vi "Sequence.FormatConditions.vi"(4 "Aliases.All":T3[](array[typedef]), 6 "Aliases Array":string[](array[string]), 8 "error in (no error)":errorcluster, 10 "Conditions":string[](array[string]), 11 "variant in":variant) -> (0 "error out":errorcluster, 1 "Warning":string, 2 "Condition":T1={"First Opreation"=enum."||", "Expression"=""}, 3 "variant out":variant)   [LabVIEW 2015, in "Simple Sequence Tools - Editor.lvlib"]
uses:
  Simple Sequence Tools - Editor.lvlib
  Shared/Types/Channel.Properties.ctl
  Types/Compiled.StepCondition.ctl
  Types/Conditions.OperationTypes.ctl
  NationalInstruments.VeriStand.RealTimeSequenceDefinitionApiUtilities
  Shared/Simple Sequence Tools - Shared.lvlib
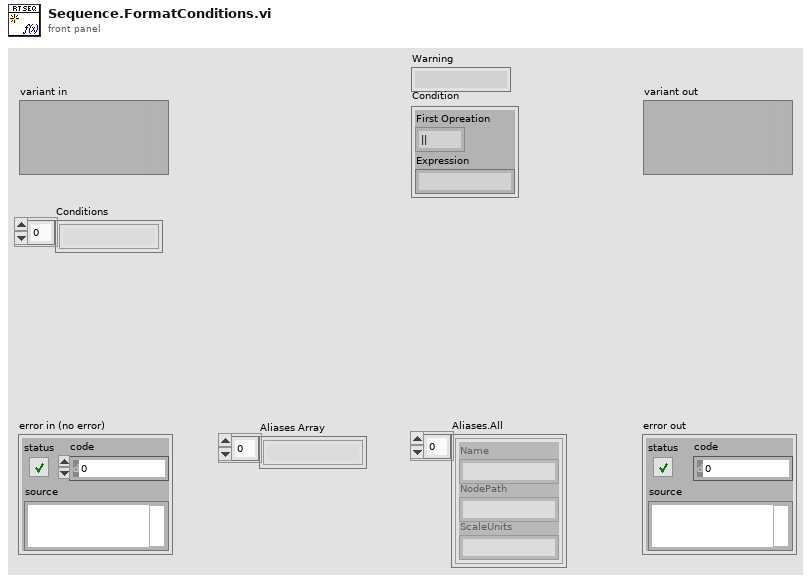
[diagram p1: front panel]
types:
  T1 = typedef "Simple Sequence Tools - Editor.lvlib/Compiled.StepCondition.ctl" = cluster{"First Opreation":T2, "Expression":string}
  T2 = typedef "Simple Sequence Tools - Editor.lvlib/Conditions.OperationTypes.ctl" = enum8{"None", "&&", "||"}
  T3 = typedef "Simple Sequence Tools - Shared.lvlib/Channel.Properties.ctl" = cluster{"Name":string, "NodePath":string, "ScaleUnits":string}
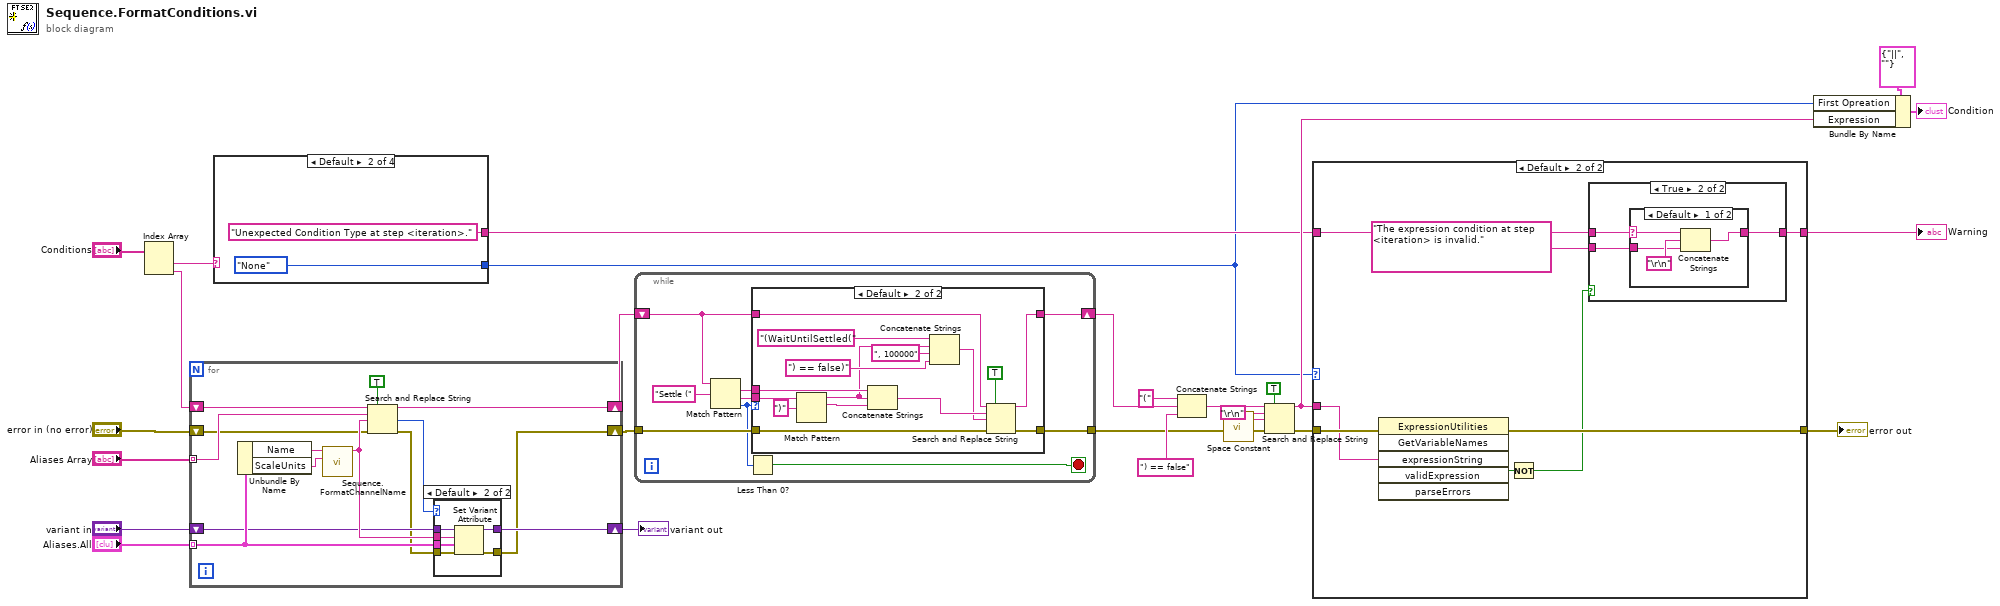
[diagram p0: block diagram]
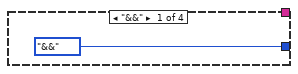
[diagram p7: hidden frame]
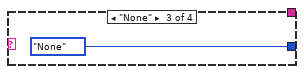
[diagram p8: hidden frame]
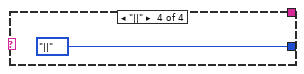
[diagram p9: hidden frame]
diagram:
  n1 = Index Array(array="Conditions") -> (element #1=w15:string, element #2=w14:string)  [unwired: 2 in]
  n2 = for {
    tunnel: "Aliases Array" -> [w40] mode=indexing
    tunnel: "Aliases.All" -> [w34] mode=indexing
    shift-right: [w27] -> w3
    shift-left: "error in (no error)" -> [w31]
    shift-right: [w35] -> w4
    shift-left: w14 -> [w39]
    shift-right: [w32] -> w26
    shift-left: "variant in" -> [w29]
    n3 = Unbundle By Name(w34) -> ("Name"=w37:string, "ScaleUnits"=w38:string)
    n4 = call "Sequence.FormatChannelName.vi"("ScaleUnits"=w38, "Name"=w37) -> ("ChannelName"=w33:string)  [unwired: 9 in]
    n5 = Search and Replace String(replace all?=TRUE ("replace all? (F)"), input string=w39, search string=w40, replace string=w33, error in=w31) -> (result string=w35:string, number of replacements=w30:i32, error out=w28:errorcluster)  [unwired: 3 in, 1 out]
    n6 = case shown="Default" w30 {
      tunnel: w34 -> [_ w48]
      tunnel: w33 -> [_ w47]
      tunnel: [w42 w46] -> w32
      tunnel: w29 -> [w42 w45]
      tunnel: w28 -> [w41 w44]
      tunnel: [w41 w43] -> w27
      frame -1, 0 {
      }
      frame Default {
        n7 = Set Variant Attribute(Variant=w45, name=w47, value=w48, error in=w44) -> (Variant out=w46:variant, error out=w43:errorcluster)  [unwired: 1 out]
      }
    }
  }
  "variant out" <- w26
  n8 = case shown="Default" w15 {
    tunnel: [Conditions.OperationTypes."&&" Conditions.OperationTypes."None" Conditions.OperationTypes."None" Conditions.OperationTypes."||"] -> w6
    tunnel: [_ "Unexpected Condition Type at step <iteration>." _ _] -> w8
    frame "&&" {
    }
    frame Default {
    }
    frame "None" {
    }
    frame "||" {
    }
  }
  n9 = while {
    shift-right: [w58] -> w1
    shift-left: w4 -> [w59]
    tunnel: w3 -> [w57]
    tunnel: [w56] -> w2
    stop <- w54 stop-if-true
    n10 = Match Pattern(string=w59, regular expression="Settle (") -> (match substring=w60:string, after substring=w61:string, offset past match=w55:i32)  [unwired: 1 in, 1 out]
    n11 = Less Than 0?(x=w55) -> (x < 0?=w54:bool)
    n12 = case shown="Default" w55 {
      tunnel: w61 -> [_ w79]
      tunnel: w60 -> [_ w74]
      tunnel: w59 -> [w64 w69]
      tunnel: [w64 w67] -> w58
      tunnel: w57 -> [w63 w66]
      tunnel: [w63 w65] -> w56
      frame -1 {
      }
      frame Default {
        n13 = Match Pattern(string=w79, regular expression=")") -> (before substring=w73:string, match substring=w72:string)  [unwired: 1 in, 2 out]
        n14 = Concatenate Strings(w74, w73, w72) -> (w71:string)
        n15 = Concatenate Strings("(WaitUntilSettled(" ("string"), w73, ", 100000" ("string"), ") == false)" ("string")) -> (w70:string)
        n16 = Search and Replace String(replace all?=TRUE ("replace all? (F)"), input string=w69, search string=w71, replace string=w70, error in=w66) -> (result string=w67:string, error out=w65:errorcluster)  [unwired: 3 in, 2 out]
      }
    }
  }
  n17 = Concatenate Strings("(" ("string"), w1, ") == false" ("string")) -> (w21:string)
  n18 = call <vilib>:"Space Constant.vi"() -> ("String"=w23:string)
  n19 = Search and Replace String(replace all?=TRUE ("replace all? (F)"), input string=w21, search string="\r\n", replace string=w23, error in=w2) -> (result string=w9:string, error out=w10:errorcluster)  [unwired: 3 in, 2 out]
  n20 = case shown="Default" w6 {
    tunnel: w10 -> [w80 w89]
    tunnel: w9 -> [_ w83]
    tunnel: w8 -> [w81 w87]
    tunnel: [w81 w86] -> w7
    tunnel: [w80 w85] -> w5
    frame "None" {
    }
    frame Default {
      n21 = invoke class="ExpressionUtilities" method="GetVariableNames"(error in=w89, "expressionString"=w83) -> (error out=w85:errorcluster, "validExpression"=w88:bool)  [unwired: 4 in, 4 out]
      n22 = Not(x=w88) -> (.not. x?=w82:bool)
      n23 = case shown="True" w82 {
        tunnel: w87 -> [w90 w92]
        tunnel: [w90 w93] -> w86
        tunnel: "The expression condition at step <iteration> is invalid." ("result string") -> [_ w91]
        frame False {
        }
        frame True {
          n24 = case shown="Default" w92 {
            selector: w92 -> [w97 _]
            tunnel: [w95 w98] -> w93
            tunnel: w91 -> [w94 w98]
            frame Default {
              n25 = Concatenate Strings(w97, "\r\n", w94) -> (w95:string)
            }
            frame "" {
            }
          }
        }
      }
    }
  }
  "Warning" <- w7
  "error out" <- w5
  n26 = Bundle By Name(cluster=T1 {"First Opreation"=enum."||", "Expression"=""} ("Condition"), "First Opreation"=w6, "Expression"=w9) -> (→"Condition":T1)
